vi "CSM Global Log Filter.vi"(7 "Cluster of class private data":T2, 11 "Cross CSM Data (in)":T3={"Name(\"\" to use uuid)"="", "Current State"="", "Arguments"="", "Source Message"={"‘State"="", "’Arguments"="", "’Error"={"status"=FALSE, "code"=0, "source"=""}}, "Source Module"="", "Complete(T)/Start(F)"=FALSE, "LogType"=enum."State Change"}) -> (0 "Matched? (dup)":bool, 3 "Cross CSM Data":T3={"Name(\"\" to use uuid)"="", "Current State"="", "Arguments"="", "Source Message"={"‘State"="", "’Arguments"="", "’Error"={"status"=FALSE, "code"=0, "source"=""}}, "Source Module"="", "Complete(T)/Start(F)"=FALSE, "LogType"=enum."State Change"})   [LabVIEW 2017]
uses:
  _Support/Typedef/_CSM_GlobalLog_MSG.ctl
  _Support/Typedef/_CSM_Response Source Message.ctl
  _Support/Typedef/_CSM_GlobalLog_MSG_TYPE.ctl
  Set Group CSM Filter.vi
  Set Group LogType Filter.vi
  Set Group State Filter.vi
  GlobalLogFilter.lvclass
  Communicable State Machine.lvlib
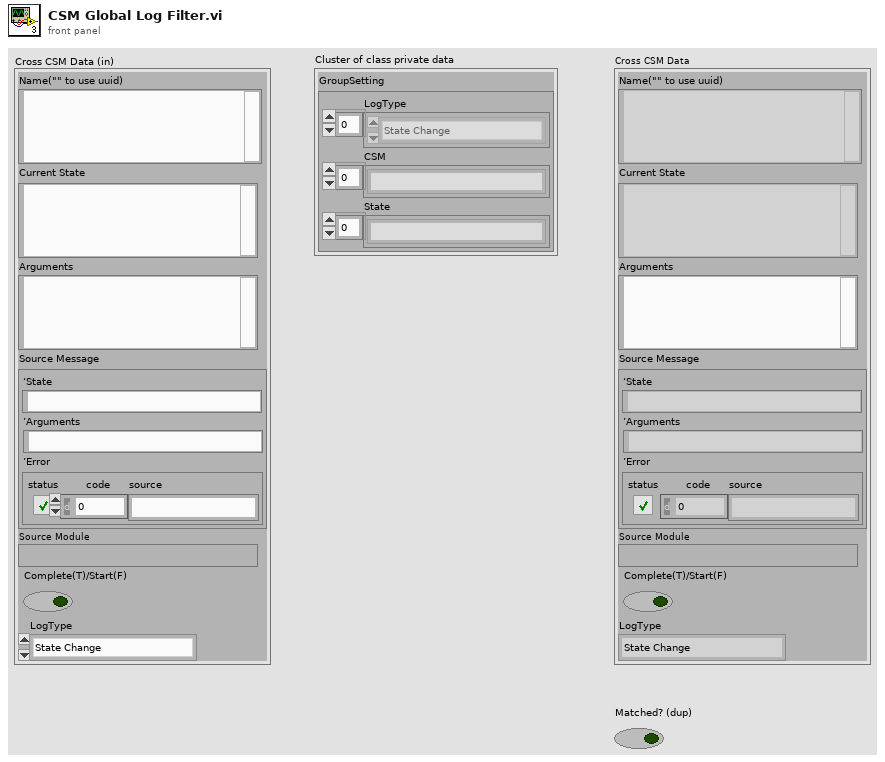
[diagram p1: front panel]
types:
  T1 = typedef "Communicable State Machine.lvlib/_CSM_GlobalLog_MSG_TYPE.ctl" = enum16{"User Log", "State Change", "Status", "Interrupt", "Register", "Unregister", "Error Log", "Module Created", "Module Destroyed"}
  T2 = cluster{"GroupSetting":cluster{"LogType":T1[], "CSM":string[], "State":string[]}}
  T3 = typedef "Communicable State Machine.lvlib/_CSM_GlobalLog_MSG.ctl" = cluster{"Name(\"\" to use uuid)":string, "Current State":string, "Arguments":string, "Source Message":T4, "Source Module":string, "Complete(T)/Start(F)":bool, "LogType":T1}
  T4 = typedef "Communicable State Machine.lvlib/_CSM_Response Source Message.ctl" = cluster{"‘State":string, "’Arguments":string, "’Error":errorcluster}
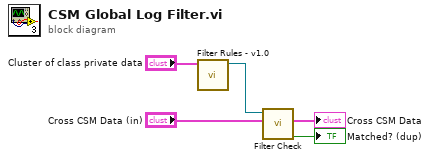
[diagram p0: block diagram]
diagram:
  n1 = call "Filter Rules - v1.0.vi"("Rules-v1"="Cluster of class private data") -> ("GlobalLogFilter out"=w3:refnum<class "GlobalLogFilter.lvclass">)  [unwired: 10 in]
  n2 = call "Filter Check.vi"("Cross CSM Data in"="Cross CSM Data (in)", "GlobalLogFilter in"=w3) -> ("Matched? (dup)"=→"Matched? (dup)":bool, "Cross CSM Data out"=→"Cross CSM Data":T3)  [unwired: 8 in]
